vi "testAcks.vi"(8 "error in (no error)":errorcluster, 11 "CoolerSerialCommand in":refnum<class "CoolerSerialCommand.lvclass">) -> (0 "error out":errorcluster, 3 "CoolerSerialCommand out":refnum<class "CoolerSerialCommand.lvclass">)   [LabVIEW 2016, in "CoolerSerialCommand.lvclass"]
uses:
  CoolerSerialCommand.lvclass
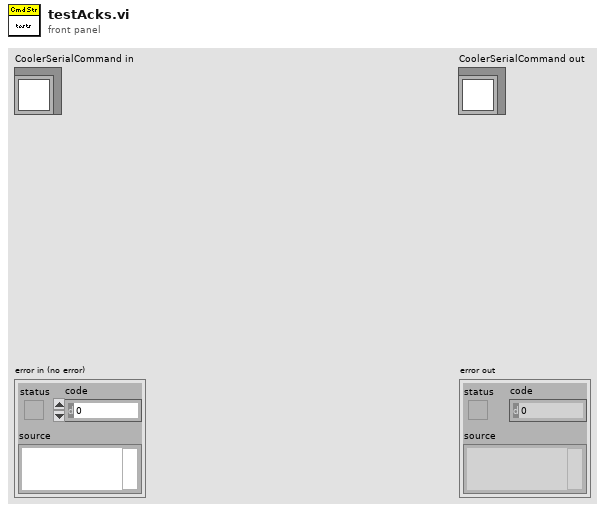
[diagram p1: front panel]
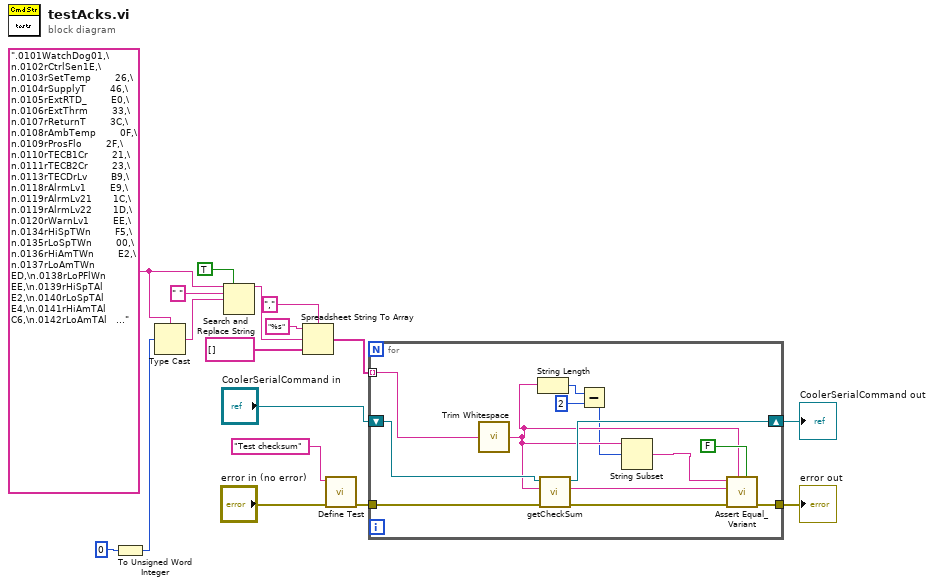
[diagram p0: block diagram]
diagram:
  w7 = ".0101WatchDog01,\n.0102rCtrlSen1E,\n.0103rSetTemp        26,\n.0104rSupplyT        46,\n.0105rExtRTD_        E0,\n.0106rExtThrm        33,\n.0107rReturnT        3C,\n.0108rAmbTemp        0F,\n.0109rProsFlo        2F,\n.0110rTECB1Cr        21,\n.0111rTECB2Cr        23,\n.0113rTECDrLv        B9,\n.0118rAlrmLv1        E9,\n.0119rAlrmLv21       1C,\n.0119rAlrmLv22       1D,\n.0120rWarnLv1        EE,\n.0134rHiSpTWn        F5,\n.0135rLoSpTWn        00,\n.0136rHiAmTWn        E2,\n.0137rLoAmTWn        ED,\n.0138rLoPFlWn        EE,\n.0139rHiSpTAl        E2,\n.0140rLoSpTAl        E4,\n.0141rHiAmTAl        C6,\n.0142rLoAmTAl        D1,\n.0143rLoPFlAl        D2,\n.0146rPulWdMo        13,\n.0148rPIDStat        E6,\n.0149rUpTime_        21,\n.0150rFanSpd1        D3,\n.0151rFanSpd2        D5,\n.0152rFanSpd3        D7,\n.0153rFanSpd4        D9,\n.0159sDUsrEEPU        1D"
  n1 = To Unsigned Word Integer(number=u16 0) -> (unsigned 16bit integer=w6:u16)
  n2 = Type Cast(type=w7, x=w6) -> (*(type *) &x=w5:string)
  n3 = Search and Replace String(replace all?=TRUE ("replace all? (F)"), input string=w7, search string=" ", replace string=w5) -> (result string=w11:string)  [unwired: 4 in, 3 out]
  n4 = Spreadsheet String To Array(delimiter (Tab)=",", format string="%s", spreadsheet string=w11, array type (2D Dbl)=string[] []) -> (array=w13:string[])
  n5 = call <vilib>:"Define Test.vi"("error in (no error)"="error in (no error)", "Label (VI Title)"="Test checksum" ("Label")) -> ("error out"=w1:errorcluster)  [unwired: 9 in]
  n6 = for {
    shift-right: [w29] -> w16
    shift-left: "CoolerSerialCommand in" -> [w30]
    tunnel: w13 -> [w27] mode=indexing
    tunnel: w1 -> [w28]
    tunnel: [w25] -> w4
    n7 = call <vilib>:"Trim Whitespace.vi"("string"=w27) -> ("trimmed string"=w21:string)  [unwired: 1 in]
    n8 = String Length(string=w21) -> (length=w20:i32)
    n9 = call "getCheckSum.vi"("error in (no error)"=w28, "response"=w21, "CoolerSerialCommand in"=w30) -> ("error out"=w26:errorcluster, "Checksum"=w24:string, "CoolerSerialCommand out"=w29:refnum<class "CoolerSerialCommand.lvclass">)  [unwired: 6 in]
    n10 = Subtract(x=w20, y=2) -> (x-y=w18:i32)
    n11 = String Subset(string=w21, offset (0)=w18) -> (substring=w22:string)  [unwired: 1 in]
    n12 = call <vilib>:"Assert Equal_Variant.vi"("Assert Only? (F)"=FALSE, "Label"=w21, "error in (no error)"=w26, "Y"=w24, "X"=w22) -> ("error out"=w25:errorcluster)  [unwired: 6 in]
  }
  "error out" <- w4
  "CoolerSerialCommand out" <- w16
